vi "XY Graph Copy Plot(s) from Clipboard.vi"(8 "error in (no error)":errorcluster, 11 "XYGraph Ref":T1) -> (0 "error out":errorcluster, 1 "Message":string, 2 "Number of Plots Added":i32)   [LabVIEW 2021, in "XY Graph Add-Ons.lvlib"]
uses:
  XY Graph Add-Ons.lvlib
  XY Graph Refnum.ctl
  746878ff-0c91-42af-a849-4f6591b29b50.vi
  XY Graph Get Plots Metadata.vi
  XY Graph Set Plots Metadata.vi
  Strings/Strings.lvlib
  Error/Error.lvlib
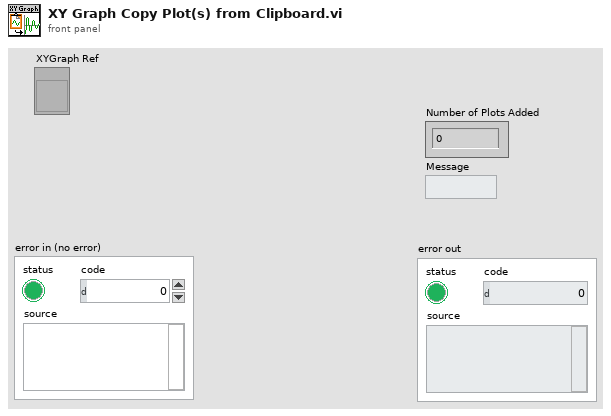
[diagram p1: front panel]
types:
  T1 = typedef "XY Graph Add-Ons.lvlib/XY Graph Refnum.ctl" = refnum<vi>
  T2 = typedef "XY Graph Add-Ons.lvlib/XY Graph Plot Format Information.ctl" = cluster{"Number of Lines to Skip":i32, "Column Header Line?":bool, "Separator":string, "Abscissa Column?":bool, "Abscissa Start":dbl, "Abscissa Step":dbl}
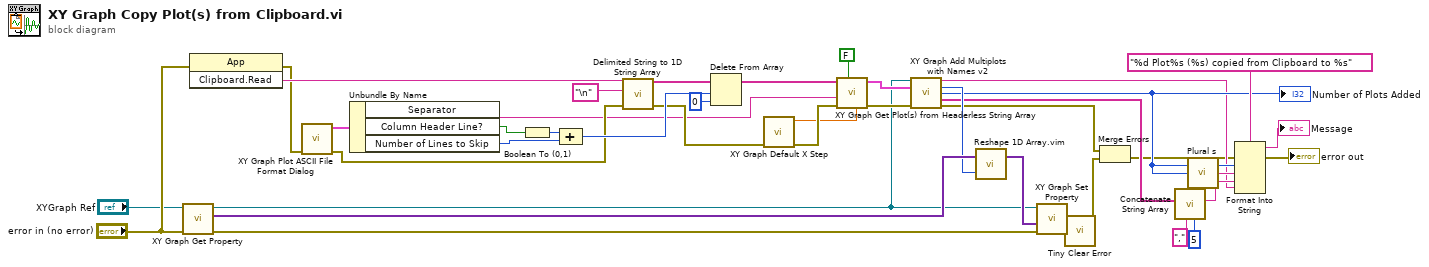
[diagram p0: block diagram]
diagram:
  n1 = call-poly "XY Graph Get Property.vi"("Error In"="error in (no error)", "XYGraph Ref"="XYGraph Ref") -> ("Error Out"=w35:errorcluster, "Plot Metadata"=w31:variant[], "XYGraph Ref (dup)"=w28:T1)  [unwired: 6 in, 1 out]
  n2 = invoke class="App" method="Clipboard.Read"(error in="error in (no error)") -> (error out=w15:errorcluster, "Read Clipbrd"=w37:string)  [unwired: 2 in, 1 out]
  n3 = call "XY Graph Plot ASCII File Format Dialog.vi"("error in (no error)"=w15) -> ("error out"=w7:errorcluster, "Plot Format Information"=w4:T2)  [unwired: 8 in, 1 out]
  n4 = Unbundle By Name(w4) -> ("Separator"=w3:string, "Column Header Line?"=w2:bool, "Number of Lines to Skip"=w1:i32)
  n5 = Boolean To (0,1)(Boolean=w2) -> (0, 1=w16:i16)
  n6 = Compound Arithmetic op=ADD(w16, w1) -> (w13:i32)
  n7 = call <vilib>:"Delimited String to 1D String Array.vi"("delimiter"="\n", "delimited string"=w37) -> ("string array"=w36:string[])  [unwired: 9 in]
  n8 = Delete From Array(array=w36, length=w13, index=0) -> (array with subset deleted=w14:string[])  [unwired: 1 out]
  n9 = call "XY Graph Default X Step.vi"("Error In"=w7) -> ("Error Out"=w6:errorcluster, "Default X Step"=w5:dbl)  [unwired: 9 in]
  n10 = call "XY Graph Get Plot(s) from Headerless String Array.vi"("Default X step (1)"=w5, "Alternating Axes?"=FALSE, "error in (no error)"=w6, "Delimiter"=w3, "Text Lines"=w14) -> ("error out"=w34:errorcluster, "Plot Array"=w33:cluster{"Array":dbl[], "Array":dbl[]}[])  [unwired: 5 in]
  n11 = call "XY Graph Add Multiplots with Names v2.vi"("XYGraph in"=w28, "Array of Plots"=w33, "error in (no error)"=w34) -> ("XY Graph Caption (or Label)"=w19:string, "Total Number of Plots"=w29:i32, "Number of Plots Added"=w25:i32, "Added Plot Names"=w21:string[], "error out"=w8:errorcluster)  [unwired: 8 in]
  "Number of Plots Added" <- w25
  n12 = call "Reshape 1D Array.vim"("dimension size"=w29, "1D Array"=w31) -> ("1D Array"=w30:variant[])  [unwired: 1 in]
  n13 = call-poly "XY Graph Set Property.vi"("error in (no error)"=w35, "Plots Metadata"=w30, "XY Graph Refnum"=w28) -> ("error out"=w27:errorcluster)  [unwired: 7 in, 1 out]
  n14 = call "Tiny Clear Error.vi"("Error In"=w27) -> ("no Error Out"=w9:errorcluster)  [unwired: 8 in]
  n15 = Merge Errors(w8, w9) -> (w10:errorcluster)
  n16 = call "Concatenate String Array.vi"("Max Number of Elements (None: -1)"=5 ("Max Number of Elements (None: 1)"), "Separator (TAB)"=",", "String Array"=w21) -> ("Formatted String"=w20:string)  [unwired: 8 in]
  n17 = call "Plural s.vi"("# Elements"=w25) -> ("Plural s"=w24:string)
  n18 = Format Into String(format string="%d Plot%s (%s) copied from Clipboard to %s", error in=w10, w25, w24, w20, w19) -> (resulting string=→"Message":string, error out=→"error out":errorcluster)  [unwired: 1 in]
